vi "Read Number of Steps.vi"(8 "error in (no error)":errorcluster, 11 "Number of Steps in":refnum<class "Number of Steps.lvclass">) -> (0 "error out":errorcluster, 2 "Number of Steps":i32, 3 "Number of Steps out":refnum<class "Number of Steps.lvclass">)   [LabVIEW 2019, in "TestEngine.lvlib" / "Number of Steps.lvclass"]
uses:
  Number of Steps.lvclass
  Number of Steps.lvclass/Number of Steps.ctl
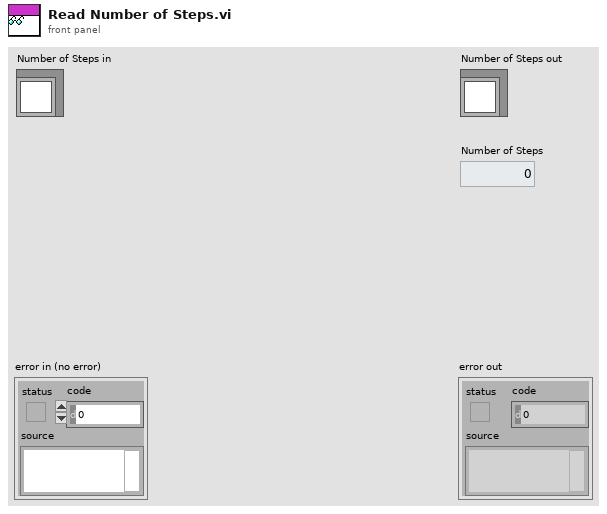
[diagram p1: front panel]
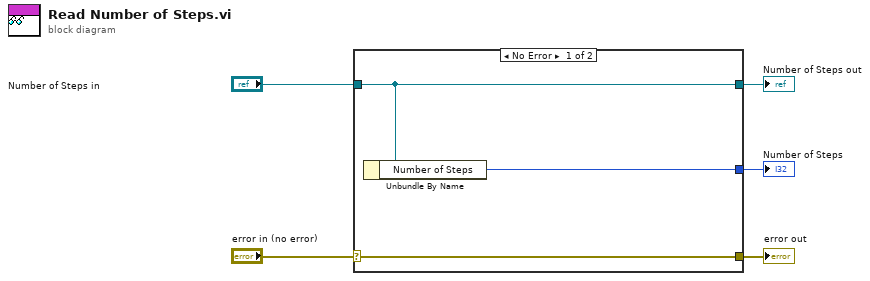
[diagram p0: block diagram]
diagram:
  n1 = case shown="No Error" "error in (no error)" {
    selector: "error in (no error)" -> [w8 w9]
    tunnel: [w8 w9] -> w4
    tunnel: [w7 w10] -> w2
    tunnel: "Number of Steps in" -> [w7 w10]
    tunnel: [w6 _] -> w1
    frame No Error {
      n2 = Unbundle By Name(w7) -> ("Number of Steps"=w6:i32)
    }
    frame Error {
    }
  }
  "error out" <- w4
  "Number of Steps out" <- w2
  "Number of Steps" <- w1
